vi "getFirstEnumName.vi"(8 "error in (no error)":errorcluster, 11 "Enumeration in":refnum<class "Enumeration.lvclass">) -> (0 "error out":errorcluster, 1 "enumListIsEmpty":bool, 2 "FirstEnumName":string, 3 "Enumeration out":refnum<class "Enumeration.lvclass">)   [LabVIEW 2018, in "Enumeration.lvclass"]
uses:
  Enumeration.lvclass
  Enumeration.lvclass/Enumeration.ctl
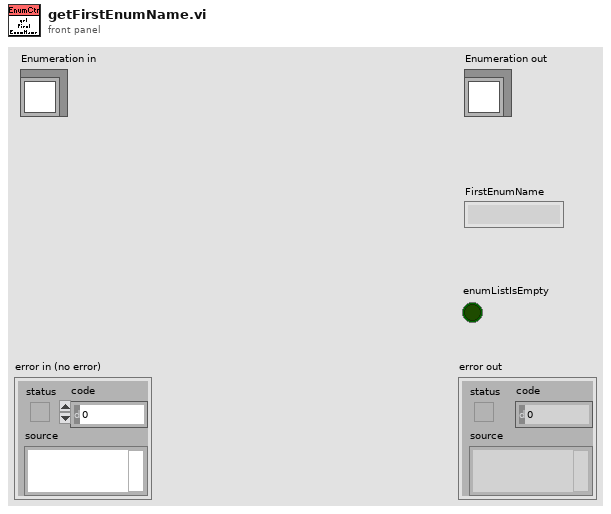
[diagram p1: front panel]
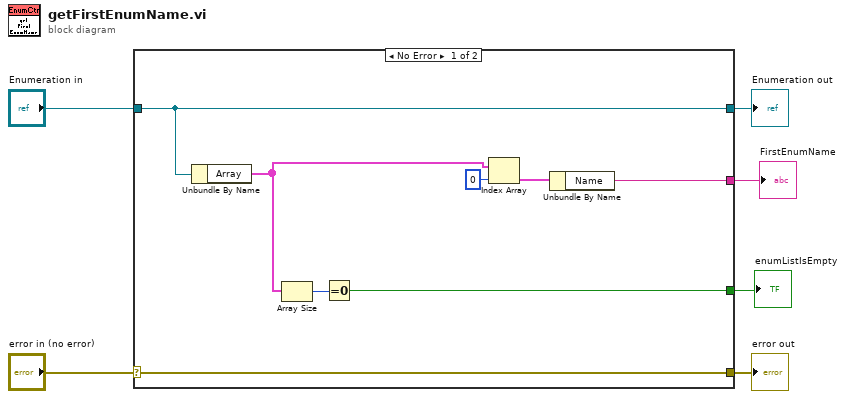
[diagram p0: block diagram]
diagram:
  n1 = case shown="No Error" "error in (no error)" {
    selector: "error in (no error)" -> [w14 w16]
    tunnel: [w14 w16] -> w5
    tunnel: [w10 w15] -> w3
    tunnel: "Enumeration in" -> [w10 w15]
    tunnel: [w11 _] -> w2
    tunnel: [w7 _] -> w1
    frame No Error {
      n2 = Unbundle By Name(w10) -> ("Array"=w9:cluster{"Name":string, "Literal":string}[])
      n3 = Array Size(array=w9) -> (size(s)=w8:i32)
      n4 = Equal To 0?(x=w8) -> (x = 0?=w7:bool)
      n5 = Index Array(array=w9, index=0) -> (element=w12:cluster{"Name":string, "Literal":string})
      n6 = Unbundle By Name(w12) -> ("Name"=w11:string)
    }
    frame Error {
    }
  }
  "error out" <- w5
  "Enumeration out" <- w3
  "FirstEnumName" <- w2
  "enumListIsEmpty" <- w1
